vi "Main.vi"(10 "Productos Subpanel":refnum<vi>, 11 "Module Admin":refnum<class "Delacor_lib_QMH_Module Admin.lvclass">) -> ()   [LabVIEW 2019, in "Products.lvlib"]
doc: "This template is based off of the Queued Message Handler design pattern and the Queued Message Handler project template that ships with LabVIEW.\n\nThe main difference is that the queue is private to this module and communication between modules is performed via Broadcast and Request events.\n\nRequest events are wrapped in public API methods and are handled in the Event Handling Loop (EHL) of this VI. Any module can register for Broadcast events sent by this module. The EHL generates messages based on user interface actions.\n\nThe Message Handling Loop (MHL) processes messages generated by the EHL, or by other messages. The messages are string values, so new messages can be added easily to the Message Cases case structure in the MHL. Each message cluster can also provide an optional value for Message Data, which is a variant that can be converted to whatever message-specific data is required.\n_____\nBased on Delacor QMH Project Template 5.0.0.82."
uses:
  Products.lvlib
  Module Data--cluster.ctl
  <vilib>/Delacor/Delacor QMH/Libraries/Message Queue_class/Delacor_lib_QMH_Message Queue.lvclass
  <vilib>/Delacor/Delacor QMH/Libraries/Message Queue_class/Delacor_lib_QMH_Enqueue Message (Single).vi
  <vilib>/ErrorRing/Error Ring.xnode
  <vilib>/Utility/error.llb/Error Cluster From Error Code.vi
  <vilib>/Delacor/Delacor QMH/Libraries/Module Admin_class/Delacor_lib_QMH_Module Admin.lvclass
  Stop Argument--cluster.ctl
  Set product Argument--cluster.ctl
  Product Selection Argument--cluster.ctl
  Mensajes/Messages.lvlib
panel:
  in  "Productos":i32(listbox)
  in  "Buy":bool
  out "error out":errorcluster
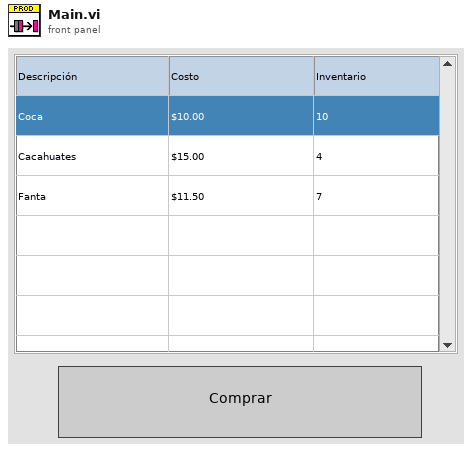
[diagram p1: front panel]
types:
  T1 = typedef "Products.lvlib/Request Events--cluster.ctl" = cluster{"Stop Module":refnum<user-event>, "Show Panel":refnum<user-event>, "Hide Panel":refnum<user-event>, "Get Module Execution Status":refnum<user-event>, "Show Diagram":refnum<user-event>, "Set product":refnum<user-event>, "Product Selection":refnum<user-event>}
  T2 = typedef "Products.lvlib/Module Data--cluster.ctl" = cluster{"Status":string, "List":i32, "List Ref":refnum<vi>, "Items":string[][], "Product selection":string[], "Numeer de producto seleccionado":i32, "Crédito":dbl}
  T3 = enum32{"invalid lock state", "Not Locked", "Locked (No Password)", "Password-protected"}
  T4 = typedef "Products.lvlib/Stop Argument--cluster.ctl" = cluster{"Origin":string, "Exit via Stop Module Req?":bool, "Wait for Module to stop?":bool}
  T5 = typedef "Products.lvlib/Set product Argument--cluster.ctl" = cluster{"Item Names":string[][]}
  T6 = typedef "Products.lvlib/Product Selection Argument--cluster.ctl" = cluster{"Product selection":i32}
  T7 = enum32{"Invalid", "Standard", "Closed", "Hidden", "Minimized", "Maximized"}
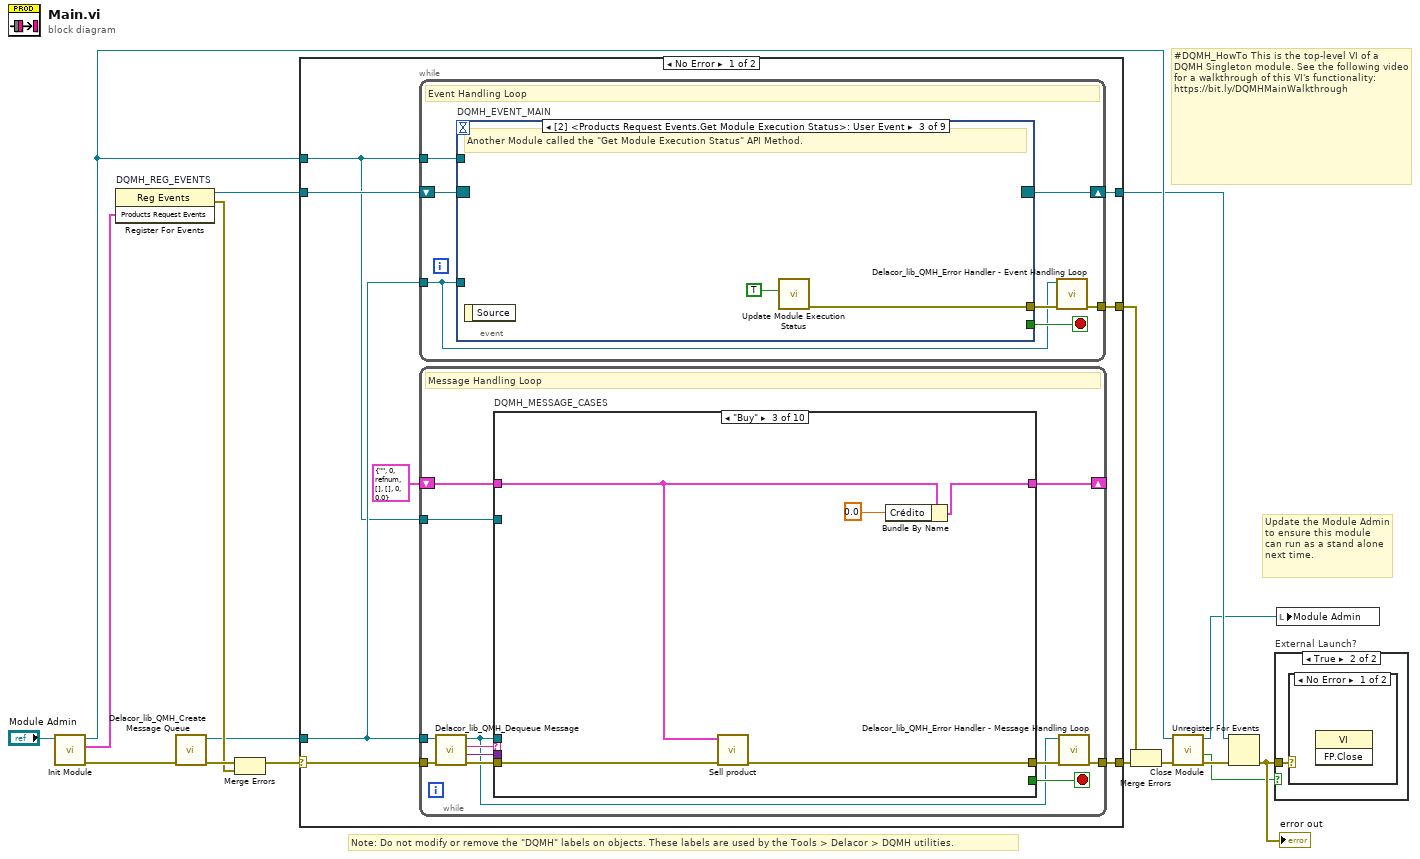
[diagram p0: block diagram]
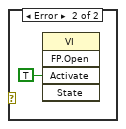
[diagram p3: hidden frame]
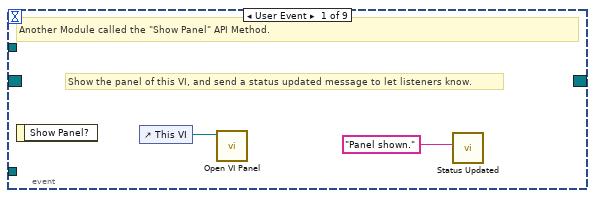
[diagram p4: hidden frame]
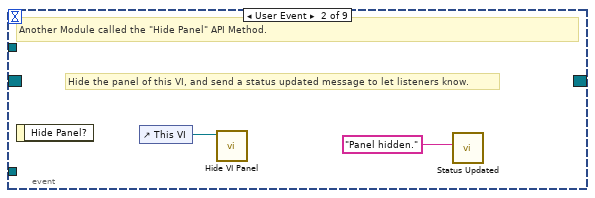
[diagram p5: hidden frame]
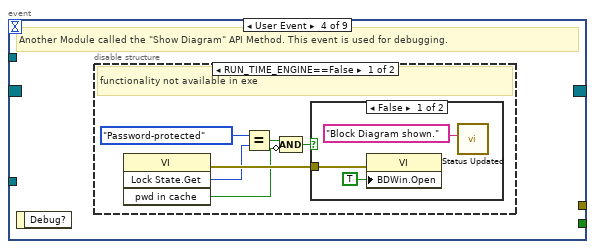
[diagram p6: hidden frame]
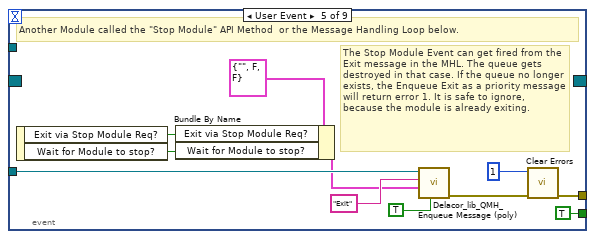
[diagram p9: hidden frame]
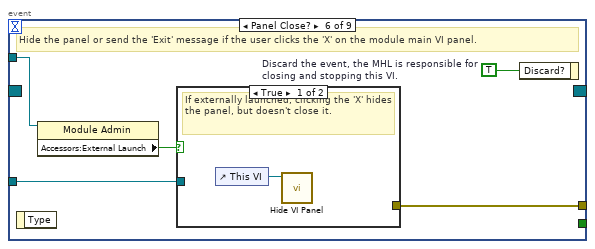
[diagram p10: hidden frame]
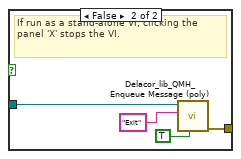
[diagram p11: hidden frame]
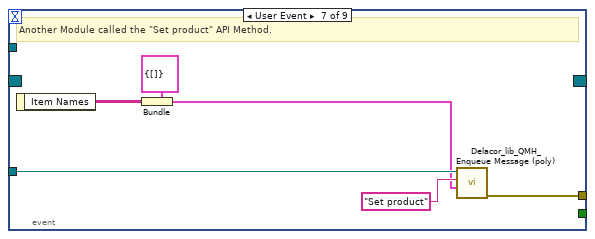
[diagram p12: hidden frame]
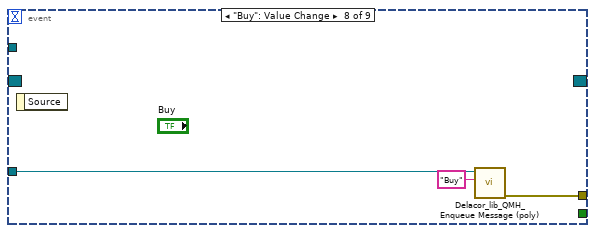
[diagram p13: hidden frame]
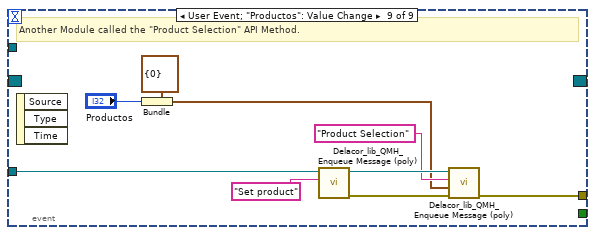
[diagram p14: hidden frame]
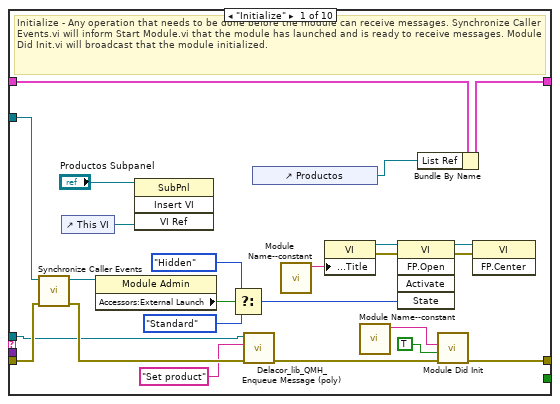
[diagram p15: hidden frame]
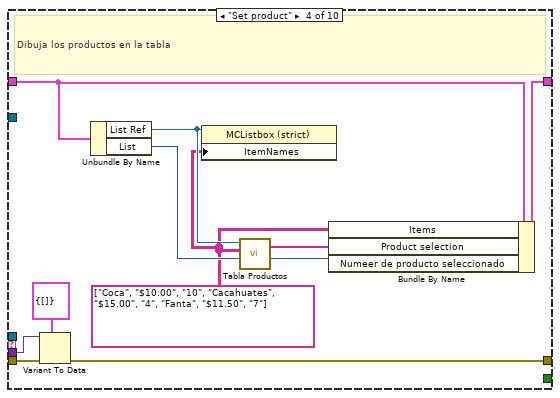
[diagram p17: hidden frame]
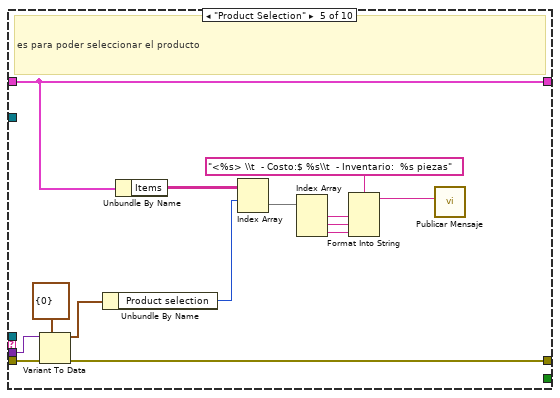
[diagram p18: hidden frame]
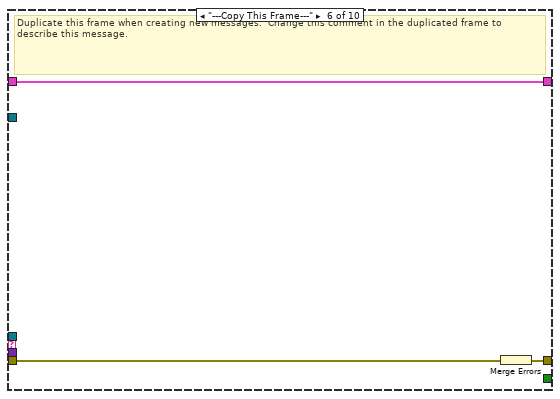
[diagram p19: hidden frame]
diagram:
  # "#DQMH_HowTo This is the top-level VI of a DQMH Singleton module. See the following video for a walkthrough of this VI's functionality: https://bit.ly/DQMHMainWalkthrough"
  # "Note: Do not modify or remove the \"DQMH\" labels on objects. These labels are used by the Tools > Delacor > DQMH utilities."
  # "Update the Module Admin to ensure this module can run as a stand alone next time."
  n1 = call "Init Module.vi"("Singleton Module Admin in"="Module Admin") -> ("error out"=w16:errorcluster, "Products Request Events"=w5:T1, "Singleton Module Admin out"=w8:refnum<class "Delacor_lib_QMH_Module Admin.lvclass">)  [unwired: 8 in]
  n2 = register-events "DQMH_REG_EVENTS"(w5) -> (reference out=w6:refnum<event-registration>, error out=w9:errorcluster)  [unwired: 2 in]
  n3 = call <vilib>:"Delacor_lib_QMH_Create Message Queue.vi"("error in (no error)"=w16) -> ("error out"=w11:errorcluster, "Message Queue"=w4:refnum<class "Delacor_lib_QMH_Message Queue.lvclass">)  [unwired: 9 in]
  n4 = Merge Errors(w11, w9) -> (w10:errorcluster)
  n5 = case shown="No Error" w10 {
    selector: w10 -> [w23 w208]
    tunnel: [w25 w207] -> w17
    tunnel: [w22 w213] -> w7
    tunnel: w6 -> [w20 w213]
    tunnel: w4 -> [w19 w206]
    tunnel: [w24 _] -> w14
    tunnel: w8 -> [w18 w209]
    frame No Error {
      n6 = while {
        tunnel: w19 -> [w26]
        shift-right: [w29] -> w22
        shift-left: w20 -> [w30]
        tunnel: [w31] -> w24
        tunnel: w18 -> [w27]
        stop <- w28 stop-if-true
        # "Event Handling Loop"
        n7 = event "DQMH_EVENT_MAIN" shown="[2] <Products Request Events.Get Module Execution Status>: User Event" {
          selector: w30 -> [_ _ _ _ _ _ _ _ _]
          dyn-events: [_ _ _ _ _ _ _ _ _] -> w29
          timeout: _ -> [_ _ _ _ _ _ _ _ _]
          tunnel: [_ _ _ _ TRUE ("Discard?") _ _ _ _] -> w28
          tunnel: w26 -> [_ _ _ _ w54 w61 w74 w77 w86]
          tunnel: [_ _ w38 _ w57 w63 w69 w75 w81] -> w32
          tunnel: w27 -> [_ _ _ _ _ w60 _ _ _]
          event User Event {
            # "Show the panel of this VI, and send a status updated message to let listeners know."
            # "Another Module called the \"Show Panel\" API Method."
            n8 = event-data() -> ()  [unwired: 1 in, 1 out]
            n9 = control-ref of="This VI"() -> (w34:refnum<vi>)
            n10 = call "Open VI Panel.vi"("VI"=w34) -> ()  [unwired: 10 in, 1 out]
            n11 = call "Status Updated.vi"("Status"="Panel shown." ("format string")) -> ()  [unwired: 10 in, 1 out]
          }
          event User Event {
            # "Hide the panel of this VI, and send a status updated message to let listeners know."
            # "Another Module called the \"Hide Panel\" API Method."
            n12 = event-data() -> ()  [unwired: 1 in, 1 out]
            n13 = control-ref of="This VI"() -> (w36:refnum<vi>)
            n14 = call "Hide VI Panel.vi"("VI"=w36) -> ()  [unwired: 10 in, 1 out]
            n15 = call "Status Updated.vi"("Status"="Panel hidden." ("format string")) -> ()  [unwired: 10 in, 1 out]
          }
          event User Event {
            # "Another Module called the \"Get Module Execution Status\" API Method."
            n16 = event-data() -> ()  [unwired: 1 in, 1 out]
            n17 = call "Update Module Execution Status.vi"("Running?"=TRUE) -> ("error out"=w38:errorcluster)  [unwired: 10 in]
          }
          event User Event {
            # "Another Module called the \"Show Diagram\" API Method. This event is used for debugging."
            n18 = event-data() -> ()  [unwired: 1 in, 1 out]
            n19 = disable-structure shown="RUN_TIME_ENGINE==False" {
              frame condition #0 (active) {
                # "functionality not available in exe"
                n20 = invoke class="VI" method="Lock State.Get"() -> (error out=w44:errorcluster, "Get Lock State"=w43:T3, "pwd in cache"=w40:bool)  [unwired: 4 in, 1 out]
                n21 = Equal?(x=T3."Password-protected", y=w43) -> (x = y?=w41:bool)
                n22 = Compound Arithmetic op=AND(w41, invert w40) -> (w39:bool)
                n23 = case shown="False" w39 {
                  tunnel: w44 -> [w47 _]
                  frame False {
                    n24 = property class="VI"(error in=w47, "BDWin.Open"=TRUE ("Block Diagram Window:Open")) -> ()  [unwired: 1 in, 2 out]
                    n25 = call "Status Updated.vi"("Status"="Block Diagram shown." ("format string")) -> ()  [unwired: 10 in, 1 out]
                  }
                  frame True {
                    # "Password-protected VI, and the password is not in the cache. Do not show the diagram."
                  }
                }
              }
              frame condition #1 {
              }
            }
          }
          event User Event {
            # "The Stop Module Event can get fired from the Exit message in the MHL. The queue gets destroyed in that case. If the queue no longer exists, the Enqueue Exit as a priority message will return error 1. It is safe to ignore, because the module is already exiting."
            # "Another Module called the \"Stop Module\" API Method  or the Message Handling Loop below."
            n26 = event-data() -> ("Exit via Stop Module Req?"=w50:bool, "Wait for Module to stop?"=w49:bool)  [unwired: 1 in]
            n27 = Bundle By Name(cluster=T4 {"Origin"="", "Exit via Stop Module Req?"=FALSE, "Wait for Module to stop?"=FALSE} ("Stop Argument"), "Exit via Stop Module Req?"=w50, "Wait for Module to stop?"=w49) -> (w48:T4)
            n28 = call-poly <vilib>:"Delacor_lib_QMH_Enqueue Message (poly).vi"("Priority Message? (F)"=TRUE, "Message Data"=w48, "Message"="Exit", "Message Queue in"=w54) -> ("error out"=w58:errorcluster)  [unwired: 6 in, 1 out]
            n29 = call <vilib>:"Clear Errors.vi"("error in (no error)"=w58, "specific error code to clear (0: all)"=1) -> ("error out"=w57:errorcluster)  [unwired: 4 in, 1 out]
          }
          event Panel Close? {
            w62 = TRUE  # Discard the event, the MHL is responsible for closing and stopping this VI.
            # "Hide the panel or send the 'Exit' message if the user clicks the 'X' on the module main VI panel."
            n30 = event-data() -> ()  [unwired: 1 in, 1 out]
            n31 = property class="Module Admin"(reference=w60) -> ("Accessors:External Launch"=w59:bool)  [unwired: 1 in, 2 out]
            n32 = case shown="True" w59 {
              tunnel: w61 -> [_ w67]
              tunnel: [_ w68] -> w63
              frame True {
                # "If externally launched, clicking the 'X' hides the panel, but doesn't close it."
                n33 = control-ref of="This VI"() -> (w64:refnum<vi>)
                n34 = call "Hide VI Panel.vi"("VI"=w64) -> ()  [unwired: 10 in, 1 out]
              }
              frame False {
                # "If run as a stand-alone VI, clicking the panel 'X' stops the VI."
                n35 = call-poly <vilib>:"Delacor_lib_QMH_Enqueue Message (poly).vi"("Priority Message? (F)"=TRUE, "Message"="Exit", "Message Queue in"=w67) -> ("error out"=w68:errorcluster)  [unwired: 7 in, 1 out]
              }
            }
            n36 = event-data("Discard?"=w62) -> ()  [unwired: 1 in, 1 out]
          }
          event User Event {
            # "Another Module called the \"Set product\" API Method."
            n37 = event-data() -> ("Item Names"=w70:string[][])  [unwired: 1 in]
            n38 = Bundle(cluster=T5 {"Item Names"=[]} ("Set product Argument"), "Item Names"=w70) -> (w71:T5)
            n39 = call-poly <vilib>:"Delacor_lib_QMH_Enqueue Message (poly).vi"("Message Data"=w71, "Message"="Set product", "Message Queue in"=w74) -> ("error out"=w69:errorcluster)  [unwired: 7 in, 1 out]
          }
          event "Buy": Value Change {
            n40 = event-data() -> ()  [unwired: 1 in, 1 out]
            n41 = call-poly <vilib>:"Delacor_lib_QMH_Enqueue Message (poly).vi"("Message"="Buy", "Message Queue in"=w77) -> ("error out"=w75:errorcluster)  [unwired: 8 in, 1 out]
          }
          event User Event; "Productos": Value Change {
            # "Another Module called the \"Product Selection\" API Method."
            n42 = event-data() -> ()  [unwired: 1 in, 3 out]
            n43 = Bundle(cluster=T6 {"Product selection"=0} ("Product Selection Argument"), "Product selection"="Productos") -> (w78:T6)
            n44 = call-poly <vilib>:"Delacor_lib_QMH_Enqueue Message (poly).vi"("Message"="Set product", "Message Queue in"=w86) -> ("error out"=w83:errorcluster, "Message Queue out"=w80:refnum<class "Delacor_lib_QMH_Message Queue.lvclass">)  [unwired: 8 in]
            n45 = call-poly <vilib>:"Delacor_lib_QMH_Enqueue Message (poly).vi"("error in (no error)"=w83, "Message Data"=w78, "Message"="Product Selection", "Message Queue in"=w80) -> ("error out"=w81:errorcluster)  [unwired: 6 in, 1 out]
          }
        }
        n46 = call-dynamic "Delacor_lib_QMH_Error Handler - Event Handling Loop.vi"("error in (no error)"=w32, "Message Queue in"=w26) -> ("dup error in"=w31:errorcluster)  [unwired: 8 in, 1 out]
      }
      n47 = while {
        tunnel: w19 -> [w89]
        shift-right: [w93] -> _
        shift-left: T2 {"Status"="", "List"=0, "List Ref"=refnum, "Items"=[], "Product selection"=[], "Numeer de producto seleccionado"=0, "Crédito"=0.0} ("Data Cluster") -> [w94]
        tunnel: w23 -> [w97]
        tunnel: [w95] -> w25
        tunnel: w18 -> [w87]
        stop <- w92 stop-if-true
        # "Message Handling Loop"
        n48 = call-dynamic "Delacor_lib_QMH_Dequeue Message.vi"("error in (no error)"=w97, "Message Queue in"=w89) -> ("error out"=w96:errorcluster, "Message Data"=w90:variant, "Message"=w91:string, "Message Queue out"=w88:refnum<class "Delacor_lib_QMH_Message Queue.lvclass">)  [unwired: 6 in]
        n49 = case "DQMH_MESSAGE_CASES" shown="\"Buy\"" w91 {
          selector: w91 -> [_ _ _ _ _ _ _ _ _ w193]
          tunnel: w88 -> [w101 _ _ _ _ _ _ w163 w185 _]
          tunnel: w96 -> [w120 w124 w129 w140 w154 w157 w159 w170 w191 w195]
          tunnel: [w118 w124 w128 w139 w153 w156 w159 w166 w188 w196] -> w98
          tunnel: w94 -> [w103 w123 w126 w136 w149 w155 w158 w165 w184 w194]
          tunnel: [w109 w123 w127 w135 w149 w155 w158 w165 w184 w194] -> w93
          tunnel: [_ _ _ _ _ _ _ _ w183 _] -> w92
          tunnel: w90 -> [_ _ _ w138 w152 _ _ w164 w182 _]
          tunnel: w87 -> [w110 _ _ _ _ _ _ w162 w177 _]
          frame "Initialize" {
            # "Initialize - Any operation that needs to be done before the module can receive messages. Synchronize Caller Events.vi will inform Start Module.vi that the module has launched and is ready to receive messages. Module Did Init.vi will broadcast that the module initialized."
            n50 = call "Synchronize Caller Events.vi"("error in (no error)"=w120, "Singleton Module Admin in"=w110) -> ("error out"=w119:errorcluster, "Singleton Module Admin out"=w106:refnum<class "Delacor_lib_QMH_Module Admin.lvclass">)  [unwired: 8 in]
            n51 = control-ref of="This VI"() -> (w105:refnum<vi>)
            n52 = property class="Module Admin"(reference=w106) -> ("Accessors:External Launch"=w114:bool)  [unwired: 1 in, 2 out]
            n53 = invoke class="SubPnl" method="Insert VI"(reference="Productos Subpanel", "VI Ref"=w105) -> ()  [unwired: 2 in, 4 out]
            n54 = Select(t=T7."Hidden" ("State"), s=w114, f=T7."Standard" ("State")) -> (s? t:f=w111:T7)
            n55 = call-poly <vilib>:"Delacor_lib_QMH_Enqueue Message (poly).vi"("error in (no error)"=w119, "Message"="Set product", "Message Queue in"=w101) -> ("error out"=w102:errorcluster)  [unwired: 7 in, 1 out]
            n56 = control-ref of="Productos"() -> (w99:refnum<vi>)
            n57 = call "Module Name--constant.vi"() -> ("Module Name"=w117:string)  [unwired: 11 in]
            n58 = property class="VI"("Front Panel.Title"=w117) -> (reference out=w116:refnum<vi>, error out=w122:errorcluster)  [unwired: 2 in]
            n59 = call "Module Name--constant.vi"() -> ("Module Name"=w107:string)  [unwired: 11 in]
            n60 = invoke class="VI" method="FP.Open"(reference=w116, error in=w122, "State"=w111) -> (reference out=w115:refnum<vi>, error out=w121:errorcluster)  [unwired: 2 in, 3 out]
            n61 = Bundle By Name(cluster=w103, "List Ref"=w99) -> (w109:T2)
            n62 = call "Module Did Init.vi"("error in (no error)"=w102, "Initialized?"=TRUE, "Origin"=w107) -> ("error out"=w118:errorcluster)  [unwired: 8 in]
            n63 = invoke class="VI" method="FP.Center"(reference=w115, error in=w121) -> ()  [unwired: 1 in, 3 out]
          }
          frame "--- Module Specific ---" {
            # "Separator -- The following cases handle messages specific to this Module."
          }
          frame "Buy" {
            n64 = call "Sell product.vi"("error in (no error)"=w129, "Data Cluster"=w126) -> ("error out"=w128:errorcluster)  [unwired: 9 in]
            n65 = Bundle By Name(cluster=w126, "Crédito"=0.0) -> (w127:T2)
          }
          frame "Set product" {
            w130 = string[][] [["Coca", "$10.00", "10"], ["Cacahuates", "$15.00", "4"], ["Fanta", "$11.50", "7"]] ("Item Names")
            # "Dibuja los productos en la tabla"
            n66 = Variant To Data(error in=w140, type=T5 {"Item Names"=[]} ("Set product Argument"), Variant=w138) -> (error out=w139:errorcluster)  [unwired: 1 out]
            n67 = Unbundle By Name(w136) -> ("List Ref"=w132:refnum<vi>, "List"=w134:i32)
            n68 = property class="MCListbox (strict)"(reference=w132, "ItemNames"=w130) -> ()  [unwired: 1 in, 2 out]
            n69 = call "Tabla Productos.vi"("Multicolumn Listbox"=w134, "Producto_precio_inventario"=w130, "Ref list"=w132) -> ("Numero Producto seleccionado"=w131:i32, "Product selection 2"=w133:string[])  [unwired: 7 in]
            n70 = Bundle By Name(cluster=w136, "Items"=w130, "Product selection"=w133, "Numeer de producto seleccionado"=w131) -> (w135:T2)
          }
          frame "Product Selection" {
            # "es para poder seleccionar el producto"
            n71 = Variant To Data(error in=w154, type=T6 {"Product selection"=0} ("Product Selection Argument"), Variant=w152) -> (data=w150:T6, error out=w153:errorcluster)
            n72 = Unbundle By Name(w150) -> ("Product selection"=w147:i32)
            n73 = Unbundle By Name(w149) -> ("Items"=w148:string[][])
            n74 = Index Array(array=w148, index (row)=w147) -> (element=w146:string[])  [unwired: 1 in]
            n75 = Index Array(array=w146) -> (element #1=w145:string, element #2=w144:string, element #3=w143:string)  [unwired: 3 in]
            n76 = Format Into String(format string="<%s> \\t  - Costo:$ %s\\t  - Inventario:  %s piezas", w145, w144, w143) -> (resulting string=w141:string)  [unwired: 2 in, 1 out]
            n77 = call "Publicar Mensaje.vi"("Mensaje"=w141) -> ()  [unwired: 10 in, 1 out]
          }
          frame "---Copy This Frame---" {
            # "Duplicate this frame when creating new messages.  Change this comment in the duplicated frame to describe this message."
            n78 = Merge Errors(w157) -> (w156:errorcluster)
          }
          frame "--- Exit and Error Handling---" {
            # "Separator - The following cases handle errors and exit messages."
          }
          frame "Error" {
            # "#CodeRecommended - If you ever change the name of this \"Error\" message, you'll need to update the name in the Check Loop Error.vi as well."
            # "#CodeRecommended - If the module is running in standalone mode (External Launch = FALSE), this code will pop up an error dialog and call the 'Exit' message if an error occurs. Add more fine-grained error handling here."
            # "Error - Check the error message data and respond accordingly. This message is sent by the \"Error Handler\" VIs at the end of each loop in this application."
            n79 = property class="Module Admin"(reference=w162) -> ("Accessors:External Launch"=w161:bool)  [unwired: 1 in, 2 out]
            n80 = Variant To Data(error in=w170, type=errorcluster {"status"=FALSE, "code"=0, "source"=""} ("error constant"), Variant=w164) -> (data=w171:errorcluster, error out=w168:errorcluster)
            n81 = call "Module Name--constant.vi"() -> ("Module Name"=w160:string)  [unwired: 11 in]
            n82 = call "Error Reported.vi"("Additional Information"=w160, "Error"=w171) -> ()  [unwired: 9 in, 1 out]
            n83 = case shown="False" w161 {
              tunnel: [w176 _] -> w167
              tunnel: w163 -> [w174 _]
              tunnel: w171 -> [w175 _]
              frame False {
                # "If the module is running standalone, then pop up an error dialog and call the \"Exit\" message."
                n84 = call <vilib>:"Simple Error Handler.vi"("error in (no error)"=w175) -> ()  [unwired: 4 in, 5 out]
                n85 = call-poly <vilib>:"Delacor_lib_QMH_Enqueue Message (poly).vi"("Priority Message? (F)"=TRUE, "Message"="Exit", "Message Queue in"=w174) -> ("error out"=w176:errorcluster)  [unwired: 7 in, 1 out]
              }
              frame True {
                # "If the module was launched externally, calling the Error Reported broadcast VI is the only action performed by the \"Error\" message. The module's caller can then process the error appropriately."
              }
            }
            n86 = Merge Errors(w168, w167) -> (w166:errorcluster)
            n87 = local write "error out"(w166) -> ()
          }
          frame "Exit" {
            w181 = 91  # 91: not all Exit messages will have an argument
            w183 = TRUE  # Stop the VI
            # "Release the message queue reference"
            # "#CodeNeeded - Add any required cleanup code here"
            # "Exit - Exit the application."
            n88 = Variant To Data(error in=w191, type=T4 {"Origin"="", "Exit via Stop Module Req?"=FALSE, "Wait for Module to stop?"=FALSE} ("Stop Argument"), Variant=w182) -> (data=w179:T4, error out=w187:errorcluster)
            n89 = call <vilib>:"Clear Errors.vi"("error in (no error)"=w187, "specific error code to clear (0: all)"=w181) -> ("error out"=w190:errorcluster)  [unwired: 4 in, 1 out]
            n90 = control-ref of="This VI"() -> (w178:refnum<vi>)
            n91 = call-dynamic "Delacor_lib_QMH_Release Message Queue.vi"("error in (no error)"=w190, "Message Queue"=w185) -> ("error out"=w189:errorcluster)  [unwired: 9 in]
            n92 = call "Handle Exit.vi"("Stop Argument"=w179, "Admin in"=w177, "VI reference"=w178) -> ("error out"=w186:errorcluster)  [unwired: 7 in, 1 out]
            n93 = Merge Errors(w189, w186) -> (w188:errorcluster)
          }
          frame Default {
            # "'Default' case only runs if there is a message that isn't defined in any of the other cases.  Output a programming error."
            n94 = call "Module Name--constant.vi"() -> ("Module Name"=w192:string)  [unwired: 11 in]
            n95 = xnode "Error Ring"("parameter 0"=w193, "parameter 1"=w192) -> ("error out"=w197:errorcluster)
            n96 = Merge Errors(w195, w197) -> (w196:errorcluster)
          }
        }
        n97 = call-dynamic "Delacor_lib_QMH_Error Handler - Message Handling Loop.vi"("error in (no error)"=w98, "Message Queue in"=w88) -> ("dup error in"=w95:errorcluster)  [unwired: 8 in, 1 out]
      }
    }
    frame Error {
      # "Synchronize Caller Events.vi will inform Start Module.vi that the module has launched and will let the code calling Start Module.vi register for broadcasts and would permit the caller receive the broadcast that an error occurred at launch time."
      n98 = call-dynamic "Delacor_lib_QMH_Release Message Queue.vi"("error in (no error)"=w208, "Message Queue"=w206) -> ("error out"=w207:errorcluster)  [unwired: 9 in]
      n99 = call "Synchronize Caller Events.vi"("Singleton Module Admin in"=w209) -> ("error out"=w214:errorcluster)  [unwired: 9 in, 1 out]
      n100 = call "Module Name--constant.vi"() -> ("Module Name"=w212:string)  [unwired: 11 in]
      n101 = Format Into String(format string="An error occurred during initialization. %s is no longer running.", w212) -> (resulting string=w210:string)  [unwired: 2 in, 1 out]
      n102 = Merge Errors(w207, w214) -> (w215:errorcluster)
      n103 = call "Error Reported.vi"("Additional Information"=w210, "Error"=w215) -> ()  [unwired: 9 in, 1 out]
    }
  }
  n104 = Merge Errors(w14, w17) -> (w13:errorcluster)
  n105 = call "Close Module.vi"("error in (no error)"=w13, "Module Admin in"=w8) -> ("error out"=w15:errorcluster, "External Launch"=w1:bool, "Module Admin out"=w2:refnum<class "Delacor_lib_QMH_Module Admin.lvclass">)  [unwired: 7 in]
  n106 = Unregister For Events(event registration refnum=w7, error in=w15) -> (error out=w12:errorcluster)
  "error out" <- w12
  n107 = case "External Launch?" shown="True" w1 {
    tunnel: w12 -> [_ w216]
    frame False {
    }
    frame True {
      n108 = case shown="No Error" w216 {
        frame No Error {
          n109 = invoke class="VI" method="FP.Close"() -> ()  [unwired: 3 in, 3 out]
        }
        frame Error {
          n110 = invoke class="VI" method="FP.Open"("Activate"=TRUE ("Activate?")) -> ()  [unwired: 4 in, 5 out]
        }
      }
    }
  }
  n111 = local write "Module Admin"(w2) -> ()
